vi "Factory (by name).vi"(0 "Obj in":refnum<class "AM.lvclass">, 7 "Class Name":string, 11 "error in (no error)":errorcluster) -> (4 "Obj out":refnum<class "AM.lvclass">, 15 "error out":errorcluster)   [LabVIEW 2015, in "AM.lvclass"]
uses:
  AM.lvclass
  AM.lvclass/AM.ctl
  SAM/SAM.lvclass
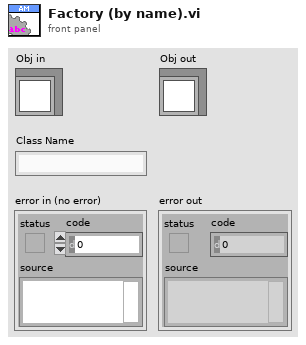
[diagram p1: front panel]
types:
  T1 = typedef "AM.lvclass/Serialized.ctl" = cluster{"Shape":enum16{"NONE", "Sinusoid", "Noise"}}
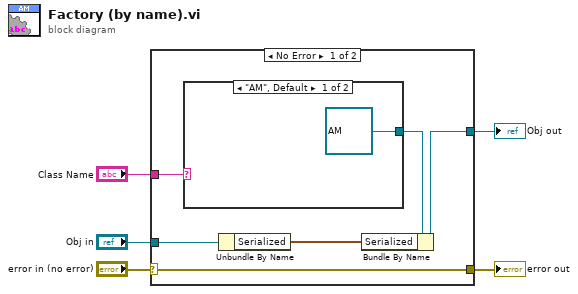
[diagram p0: block diagram]
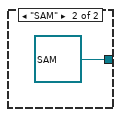
[diagram p2: hidden frame]
diagram:
  n1 = case shown="No Error" "error in (no error)" {
    selector: "error in (no error)" -> [w9 w15]
    tunnel: [w9 w15] -> w4
    tunnel: [w7 w14] -> w2
    tunnel: "Obj in" -> [w8 w14]
    tunnel: "Class Name" -> [w10 _]
    frame No Error {
      n2 = case shown="\"AM\", Default" w10 {
        tunnel: [refnum<class "AM.lvclass"> refnum ("AM") refnum<class "SAM.lvclass"> refnum ("SAM")] -> w11
        frame "AM", Default {
        }
        frame "SAM" {
        }
      }
      n3 = Unbundle By Name(w8) -> ("Serialized"=w6:T1)
      n4 = Bundle By Name(cluster=w11, "Serialized"=w6) -> (w7:refnum<class "AM.lvclass">)
    }
    frame Error {
    }
  }
  "error out" <- w4
  "Obj out" <- w2
